vi "FTW-Example-ProducerConsumerSockets.vi"() -> ()   [LabVIEW 2015]
uses:
  source/actor/Message/Base/FTW-Message.lvclass
  source/actor/Ether/FTW-Ether.lvclass
  source/actor/Producer/FTW-Producer.lvclass
  source/actor/Consumer/FTW-Consumer.lvclass
panel:
  out "Sender Identity":string
  out "Elapsed Time":dbl format="%.6fsec"
  in  "Connection":string(combo)="inproc://*"
  out "Sender Body":string
  out "Sender Header":string
  out "Timed out?":bool
  out "Actual Server Address":string
  out "error out":errorcluster
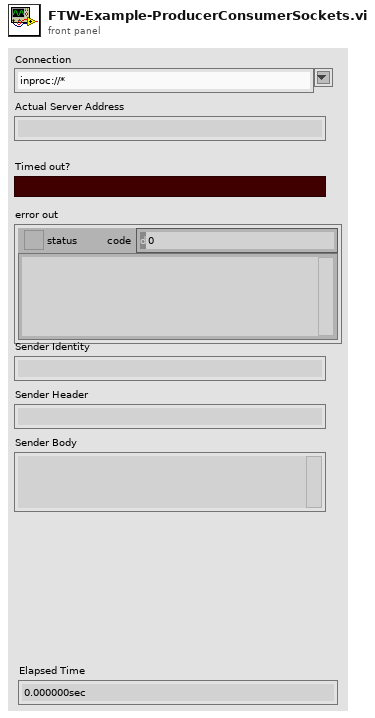
[diagram p1: front panel]
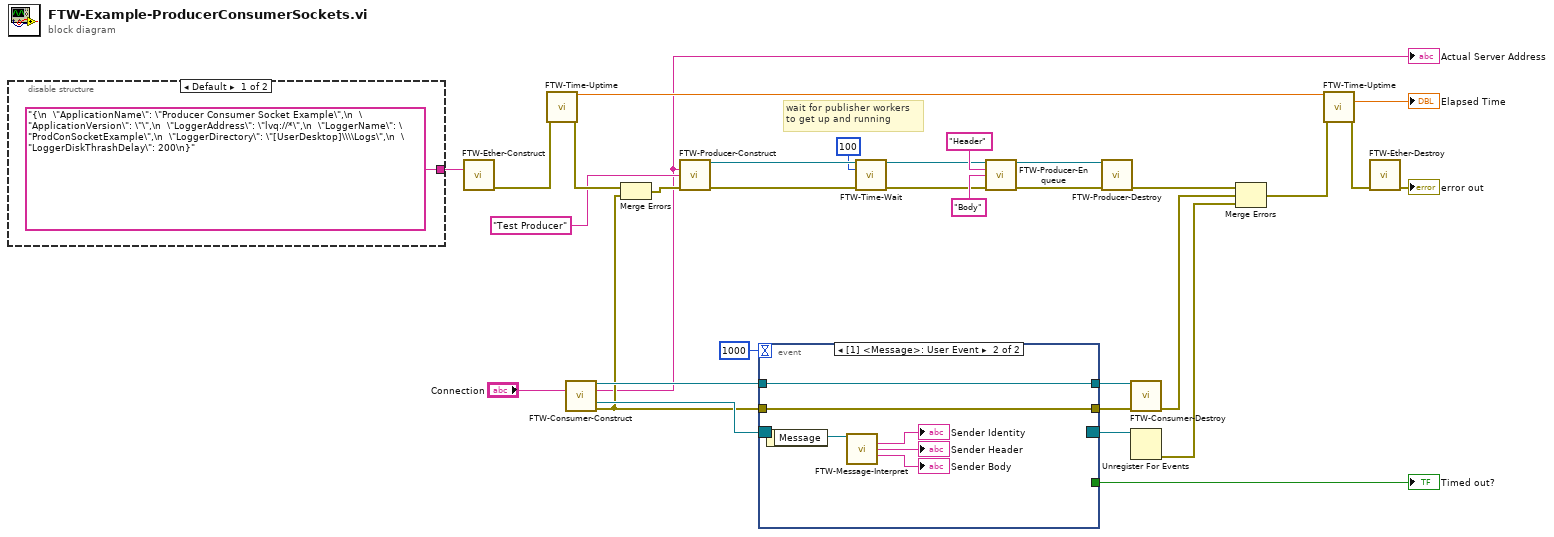
[diagram p0: block diagram]
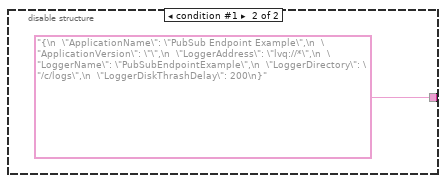
[diagram p2: hidden frame]
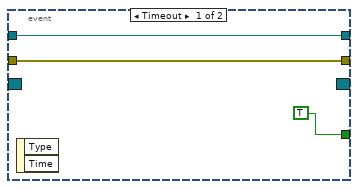
[diagram p3: hidden frame]
diagram:
  # "wait for publisher workers\nto get up and running"
  n1 = disable-structure shown="Default" {
    disable-tunnel: ["{\n  \"ApplicationName\": \"Producer Consumer Socket Example\",\n  \"ApplicationVersion\": \"\",\n  \"LoggerAddress\": \"lvq://*\",\n  \"LoggerName\": \"ProdConSocketExample\",\n  \"LoggerDirectory\": \"[UserDesktop]\\\\Logs\",\n  \"LoggerDiskThrashDelay\": 200\n}" ("FTW Ether Configuration") "{\n  \"ApplicationName\": \"PubSub Endpoint Example\",\n  \"ApplicationVersion\": \"\",\n  \"LoggerAddress\": \"lvq://*\",\n  \"LoggerName\": \"PubSubEndpointExample\",\n  \"LoggerDirectory\": \"/c/logs\",\n  \"LoggerDiskThrashDelay\": 200\n}" ("FTW Ether Configuration")] -> w29
    frame condition #0 (active) {
    }
    frame condition #1 {
    }
  }
  n2 = call "FTW-Ether-Construct.vi"("FTW Ether Configuration"=w29) -> ("error out"=w27:errorcluster)  [unwired: 14 in]
  n3 = call "FTW-Time-Uptime.vi"("error in"=w27) -> ("Current Uptime"=w10:dbl, "error out"=w11:errorcluster)  [unwired: 12 in, 1 out]
  n4 = call "FTW-Consumer-Construct.vi"("Address"="Connection") -> ("FTW-Consumer Out"=w25:refnum<class "FTW-Consumer.lvclass">, "Actual Address"=w1:string, "Event Registration Refnum"=w26:refnum<event-registration>, "error out"=w5:errorcluster)  [unwired: 11 in]
  "Actual Server Address" <- w1
  n5 = Merge Errors(w11, w5) -> (w7:errorcluster)
  n6 = call "FTW-Producer-Construct.vi"("Server Address"=w1, "Identity"="Test Producer", "error in"=w7) -> ("FTW-Producer Out"=w24:refnum<class "FTW-Producer.lvclass">, "error out"=w23:errorcluster)  [unwired: 11 in]
  n7 = event shown="[1] <Message>: User Event" {
    selector: w26 -> [_ _]
    dyn-events: [_ _] -> w14
    timeout: 1000 -> [_ _]
    tunnel: w25 -> [w36 w41]
    tunnel: w5 -> [w35 w40]
    tunnel: [w36 w41] -> w22
    tunnel: [w35 w40] -> w21
    tunnel: [TRUE _] -> w15
    event Timeout {
      n8 = event-data() -> ()  [unwired: 1 in, 2 out]
    }
    event User Event {
      n9 = event-data() -> ("Message"=w42:refnum<class "FTW-Message.lvclass">)  [unwired: 1 in]
      n10 = call-dynamic "FTW-Message-Interpret.vi"("FTW Message"=w42) -> ("Sender Identity"=→"Sender Identity":string, "Message Header"=→"Sender Header":string, "Message Body"=→"Sender Body":string)  [unwired: 10 in, 2 out]
    }
  }
  "Timed out?" <- w15
  n11 = call "FTW-Time-Wait.vi"("Wait Time (ms)"=u32 100, "error in"=w23) -> ("error out"=w17:errorcluster)  [unwired: 13 in]
  n12 = call "FTW-Producer-Enqueue.vi"("FTW-Producer In"=w24, "Header"="Header" ("Message Header"), "Body"="Body" ("Message Body"), "error in"=w17) -> ("FTW-Producer Out"=w19:refnum<class "FTW-Producer.lvclass">, "error out"=w4:errorcluster)  [unwired: 8 in, 2 out]
  n13 = call "FTW-Producer-Destroy.vi"("FTW-Producer In"=w19, "error in"=w4) -> ("error out"=w3:errorcluster)  [unwired: 13 in]
  n14 = call "FTW-Consumer-Destroy.vi"("FTW-Consumer In"=w22, "error in"=w21) -> ("error out"=w20:errorcluster)  [unwired: 13 in]
  n15 = Unregister For Events(event registration refnum=w14) -> (error out=w13:errorcluster)  [unwired: 1 in]
  n16 = Merge Errors(w3, w20, w13) -> (w2:errorcluster)
  n17 = call "FTW-Time-Uptime.vi"("Previous Uptime"=w10, "error in"=w2) -> ("Elapsed Time"=→"Elapsed Time":dbl, "error out"=w12:errorcluster)  [unwired: 11 in, 1 out]
  n18 = call "FTW-Ether-Destroy.vi"("error in"=w12) -> ("error out"=→"error out":errorcluster)  [unwired: 14 in]
